vi "DAQmx_Digital(false).vi"(8 "Error in":errorcluster, 10 "Data":bool[](array[boolean]), 11 "lines":tag caption="Line") -> (3 "Error out":errorcluster)   [LabVIEW 2011]
panel:
  in  "Name to assign":string="NI6509"
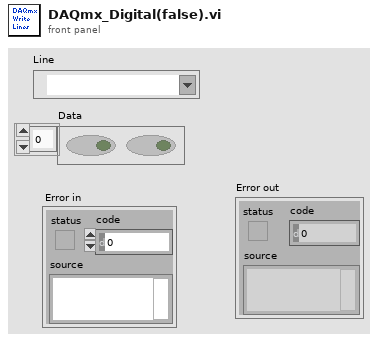
[diagram p1: front panel]
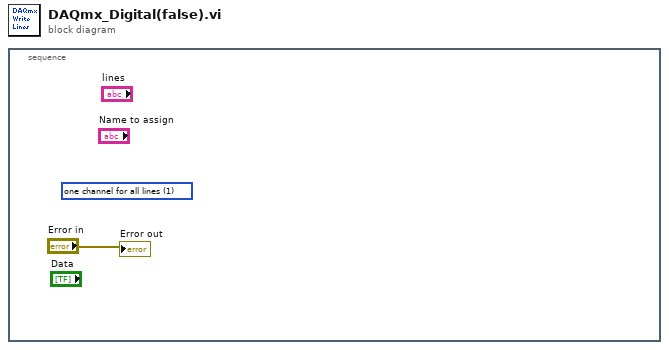
[diagram p0: block diagram]
diagram:
  n1 = stacked-sequence {
    frame #0 {
      (unwired) 1 items=["one channel for each line", "one channel for all lines", ""] ("line grouping")
      "Error out" <- "Error in"
    }
  }
